vi "Compressor Thing.vi"   [LabVIEW 2014]
uses:
  <vilib>/Rock Robotics/WPI/Solenoid/WPI_SolenoidOpenSingle.vi
  <vilib>/Rock Robotics/WPI/Solenoid/WPI_SolenoidChannel.ctl
  <vilib>/Rock Robotics/WPI/Solenoid/WPI_SolenoidSetEnum.vi
types:
  T1 = typedef "WPI_SolenoidChannel.ctl" = enum8{"Solenoid 0", "Solenoid 1", "Solenoid 2", "Solenoid 3", "Solenoid 4", "Solenoid 5", "Solenoid 6", "Solenoid 7", "Invalid"}
  T2 = typedef "WPI_SolenoidDevRef.ctl" = cluster{"DevStatus":errorcluster, "Pneumatics Control Module":u8, "Forward Solenoid Channel":T1, "Reverse Solenoid Channel":T1}
  T3 = typedef "WPI_CompressorDevRef.ctl" = cluster{"DevStatus":errorcluster, "Pneumatics Control Module":u8}
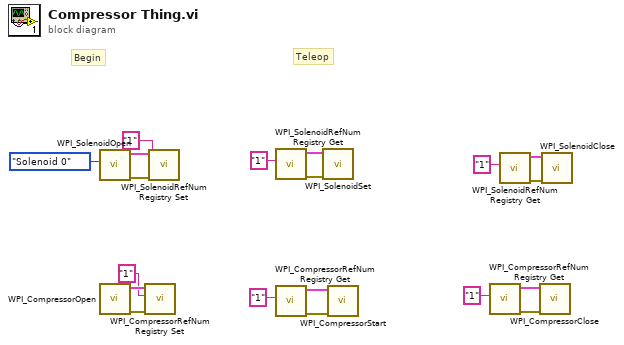
[diagram p0: block diagram]
diagram:
  # "Teleop"
  # "Begin"
  n1 = call-poly <vilib>:"WPI_SolenoidOpen.vi"("Solenoid Channel"=WPI_SolenoidChannel."Solenoid 0") -> ("error out"=w18:errorcluster, "SolenoidDevRef"=w17:T2)  [unwired: 9 in]
  n2 = call <vilib>:"WPI_CompressorOpen.vi"() -> ("CompressorDevRef"=w8:T3, "error out"=w9:errorcluster)  [unwired: 14 in]
  n3 = call <vilib>:"WPI_CompressorRefNum Registry Set.vi"("error in (no error)"=w9, "refnum name"="1", "CompressorDevRef"=w8) -> ()  [unwired: 7 in, 2 out]
  n4 = call <vilib>:"WPI_SolenoidRefNum Registry Set.vi"("error in (no error)"=w18, "refnum name"="1", "SolenoidDevRef"=w17) -> ()  [unwired: 7 in, 2 out]
  n5 = call <vilib>:"WPI_SolenoidRefNum Registry Get.vi"("refnum name"="1") -> ("error out"=w11:errorcluster, "SolenoidDevRef"=w10:T2)  [unwired: 9 in]
  n6 = call <vilib>:"WPI_CompressorRefNum Registry Get.vi"("refnum name"="1") -> ("error out"=w6:errorcluster, "CompressorDevRef"=w5:T3)  [unwired: 9 in]
  n7 = call-poly <vilib>:"WPI_SolenoidSet.vi"("error in (no error)"=w11, "SolenoidDevRef"=w10) -> ()  [unwired: 8 in, 2 out]
  n8 = call <vilib>:"WPI_CompressorStart.vi"("error in (no error)"=w6, "CompressorDevRef"=w5) -> ()  [unwired: 8 in, 2 out]
  n9 = call <vilib>:"WPI_CompressorRefNum Registry Get.vi"("refnum name"="1") -> ("error out"=w3:errorcluster, "CompressorDevRef"=w2:T3)  [unwired: 9 in]
  n10 = call <vilib>:"WPI_SolenoidRefNum Registry Get.vi"("refnum name"="1") -> ("error out"=w14:errorcluster, "SolenoidDevRef"=w13:T2)  [unwired: 9 in]
  n11 = call <vilib>:"WPI_CompressorClose.vi"("error in (no error)"=w3, "CompressorDevRef"=w2) -> ()  [unwired: 9 in, 1 out]
  n12 = call <vilib>:"WPI_SolenoidClose.vi"("error in (no error)"=w14, "SolenoidDevRef"=w13) -> ()  [unwired: 9 in, 1 out]
